vi "V-Meter Adjust Measure.vi"(6 "error in (no error)":errorcluster, 9 "VISA resource name in":refnum<visa-resource-name>) -> (0 "error out":errorcluster, 3 "VISA resource name out":refnum<visa-resource-name>)   [LabVIEW 2016, in "Hall Effect Library.lvlib"]
uses:
  Hall Effect Library.lvlib
  Global Variables/Instruments.vi
  Global Variables/Test Settings.vi
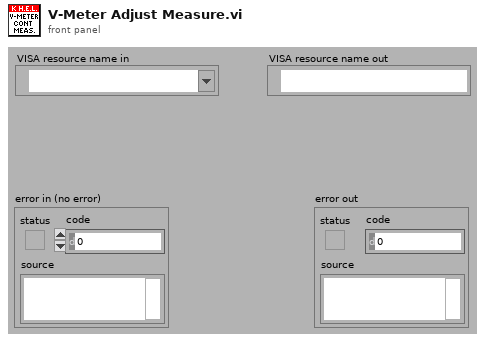
[diagram p1: front panel]
types:
  T1 = typedef "Hall Effect Library.lvlib/Voltmeters.ctl" = enum16{"2000", "2182A", "3706A"}
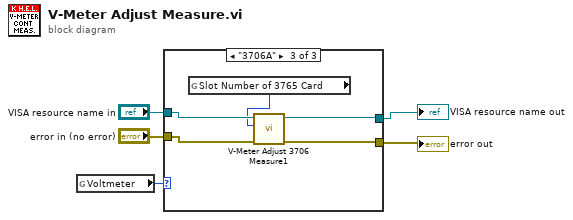
[diagram p0: block diagram]
diagram:
  n1 = global read "Instruments.vi" "Voltmeter"() -> (w5:T1)
  n2 = case shown="\"3706A\"" w5 {
    tunnel: "error in (no error)" -> [w6 w8 w13]
    tunnel: "VISA resource name in" -> [w7 w9 w14]
    tunnel: [w7 w9 w11] -> w2
    tunnel: [w6 w8 w10] -> w1
    frame "2000" {
    }
    frame "2182A", Default {
    }
    frame "3706A" {
      n3 = global read "Test Settings.vi" "Slot Number of 3765 Card"() -> (w12:u32)
      n4 = call "V-Meter Adjust 3706 Measure1.vi"("error in (no error)"=w13, "Slot Number"=w12, "VISA resource name in"=w14) -> ("error out"=w10:errorcluster, "VISA resource name out"=w11:refnum<visa-resource-name>)  [unwired: 7 in]
    }
  }
  "error out" <- w1
  "VISA resource name out" <- w2
